vi "qTPC.vi"(0 "System no.":i32=1 min=1 max=4 step=1, 5 "error in":errorcluster) -> (14 "Number of piezo channels":i32, 19 "error out":errorcluster)   [LabVIEW 2020]
doc: "Returns the number of available piezo channels. \n\nE-517, E-518: Using the Sensor Enable parameter, ID 0x02000000, you can change the controller configuration in case of hardware changes, e.g. if you install additional sensor and/or amplifier channels in the system. If this parameter is changed, the Number Of Piezo Channels parameter is adapted automatically.E.g.if parameter 0x02000000 is set to \"disabled\" for a sensor channel, thecorresponding piezo channel is disabled too and no longer included in the TPC? response. See \"Configure Axes and Channels\" in the controller user manual for details.\n\nE-709, E-712, E-725, E-727: Returns all Output Signal Channels (piezo channels + analog output channels)."
panel:
  # "Returns the number of available piezo channels."
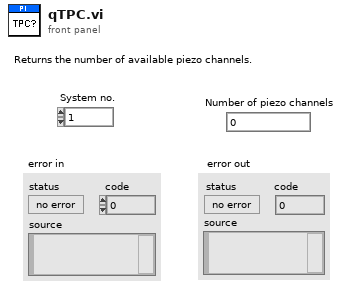
[diagram p1: front panel]
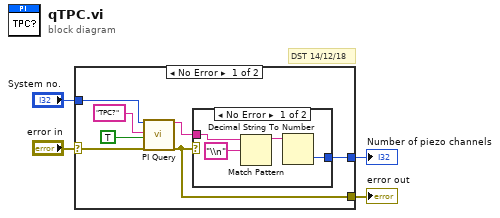
[diagram p0: block diagram]
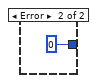
[diagram p2: hidden frame]
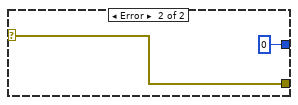
[diagram p3: hidden frame]
diagram:
  # "DST 14/12/18"
  n1 = case shown="No Error" "error in" {
    selector: "error in" -> [w5 w18]
    tunnel: [w11 0] -> w4
    tunnel: "System no." -> [w9 _]
    tunnel: [w6 w18] -> w2
    frame No Error {
      n2 = call "PI Query.vi"("System no."=w9, "String to send"="TPC?", "Attach termination char.?"=TRUE ("Attach Linefeed?"), "error in"=w5) -> ("String read"=w7:string, "error out"=w6:errorcluster)  [unwired: 3 in, 11 out]
      n3 = case shown="No Error" w6 {
        tunnel: w7 -> [w14 _]
        tunnel: [w15 0] -> w11
        frame No Error {
          n4 = Match Pattern(string=w14, regular expression="\\n") -> (before substring=w12:string)  [unwired: 4 out]
          n5 = Decimal String To Number(string=w12) -> (number=w15:i32)  [unwired: 3 out]
        }
        frame Error {
        }
      }
    }
    frame Error {
    }
  }
  "error out" <- w2
  "Number of piezo channels" <- w4
